vi "RunTest.vi"(8 "error in":errorcluster, 11 "Prueba31 in":refnum<class "Prueba031.lvclass">) -> (0 "error out":errorcluster, 2 "Resultado":string, 3 "Prueba31 out":refnum<class "Prueba031.lvclass">)   [LabVIEW 2019, in "Prueba031.lvclass"]
uses:
  Prueba031.lvclass
  Prueba031.lvclass/Prueba031.ctl
  <vilib>/Utility/miscctls.llb/LVRowAndColumnTypeDef.ctl
  QMH/Message Queue/Enqueue Message (Single).vi
  <vilib>/Utility/error.llb/Error Cluster From Error Code.vi
  RerenceAllControlsToolkit/_get control reference by name.vi
  <vilib>/ErrorRing/Error Ring.xnode
  QMH/Message Queue/Message Queue.lvlib
  QMH/User Event - Stop/User Event - Stop.lvlib
panel:
  in  "Tab":enum32{"externo", "interno"}(tab)
  out "Pict RingB_Ext":u16(ring)
  out "curva_referencia_Ext":dbl
  in  "cb_frec_Ext":string(combo)="63"
  in  "boton_generar_Ext":bool
  out "cumple_Ext":bool
  out "no_cumple_Ext":bool
  in  "seguir_Ext":bool
  out "voltaje_Ext":dbl format="%_3f"
  out "frecuencia_Ext":dbl format="%.2f"
  out "tipo generador_Ext":string
  out "Pict RingA_Ext":u16(ring)
  in  "Tabla_Ext":string[][](table)=[["63"], ["125"], ["250"], ["500"], ["1000"], ["2000"], ["4000"], ["8000"]]
  out "cumple_Int":bool
  out "no_cumple_Int":bool
  in  "seguir_Int":bool
  out "tipo generador_Int":string
  out "Pict RingA_Int":u16(ring)
  out "Pict RingB_Int":u16(ring)
  in  "Tabla_Int":string[][](table)
  # "Vienen de base de datos\nambos\ncambiar a numerico indicador"
  # "Cumple"
  # "No Cumple"
  # "Ponderación C"
  # "Curva de Referencia"
  # "Frecuencia"
  # "3. Ensayo con ponderación frecuencial C con señales acústicas. IEC 61672-3:2006 Cláusula 11"
  # "Monitoreo"
  # "Frecuencia"
  # "Hz"
  # "Voltaje"
  # "V"
  # "Cumple"
  # "No Cumple"
  # "Ponderación C"
  # "3. Ensayo con ponderación frecuencial C con señales acústicas. IEC 61672-3:2006 Cláusula 11"
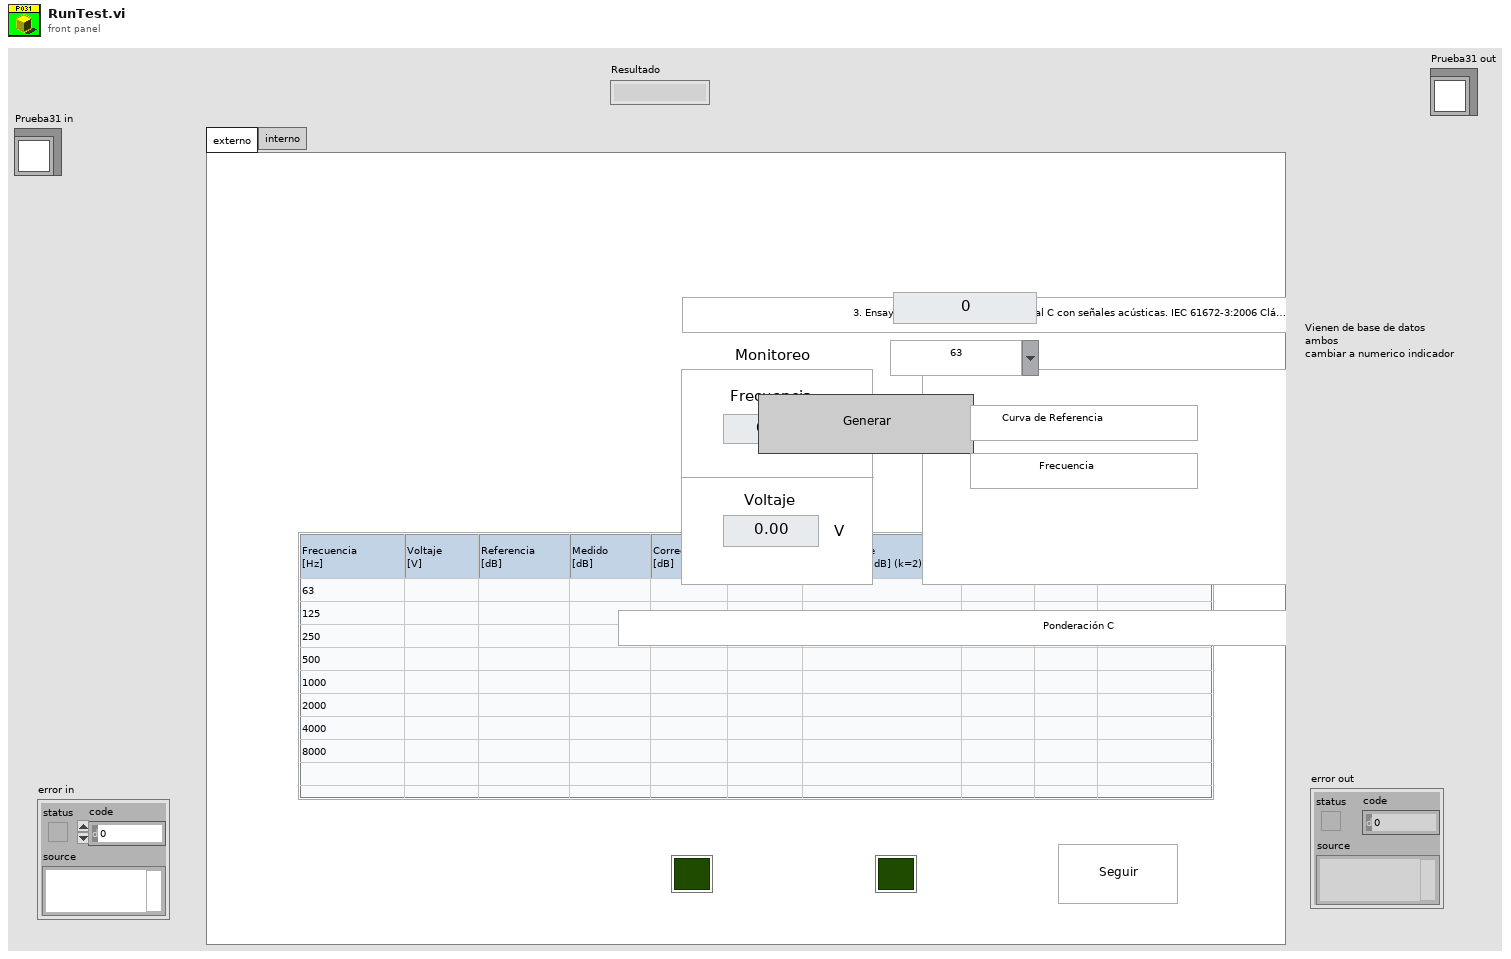
[diagram p1: front panel]
types:
  T1 = typedef "Message Queue.lvlib/All Message Queues.ctl" = cluster{"MHL":refnum<queue>, "Inst_CNT90":refnum<queue>, "Inst_DS360":refnum<queue>, "Inst_Keithley2002":refnum<queue>, "Inst_DAQ":refnum<queue>, "BD":refnum<queue>, "Pistofono":refnum<queue>, "Nexus":refnum<queue>}
  T2 = typedef "LVRowAndColumnTypeDef.ctl" = cluster{"Row":i32, "Column":i32}
  T3 = cluster{"ControlName":string, "ControlReference":refnum<vi>}[]
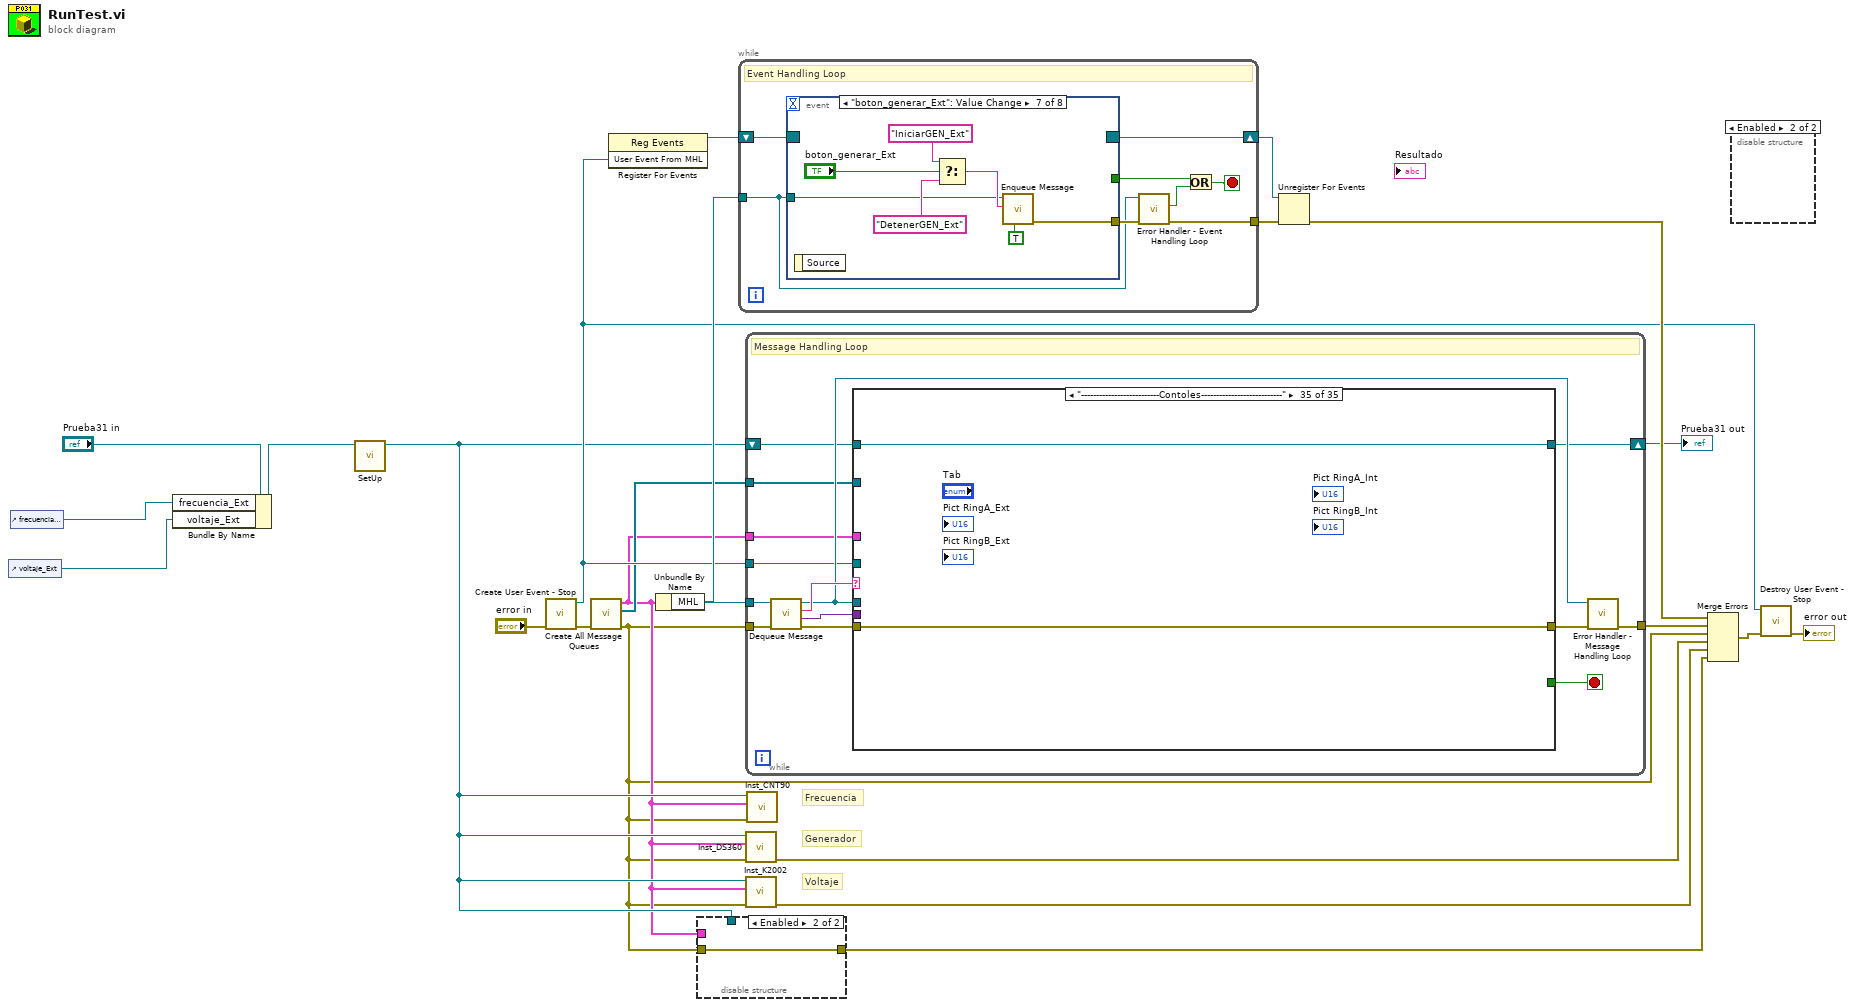
[diagram p0: block diagram]
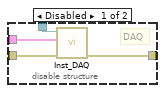
[diagram p2: hidden frame]
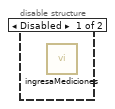
[diagram p3: hidden frame]
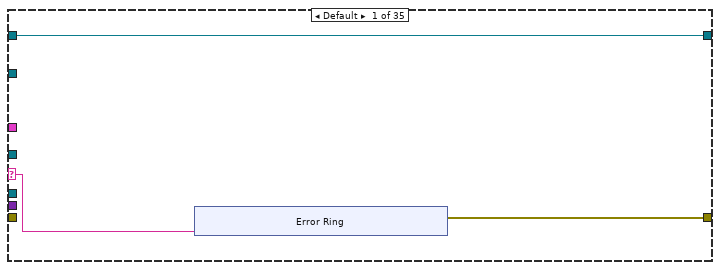
[diagram p4: hidden frame]
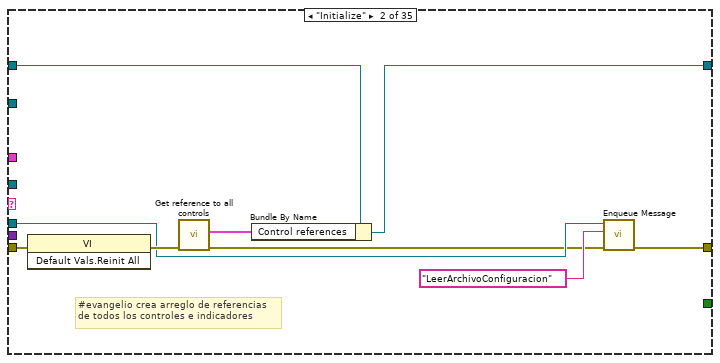
[diagram p5: hidden frame]
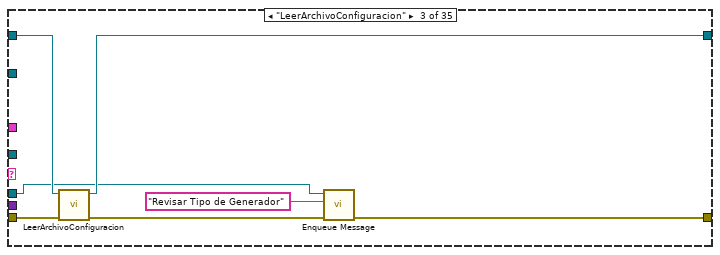
[diagram p6: hidden frame]
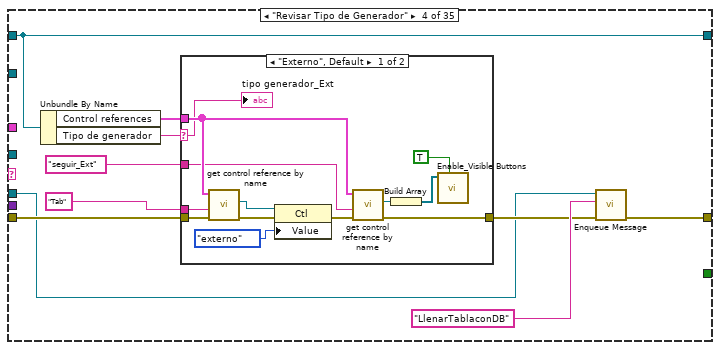
[diagram p7: hidden frame]
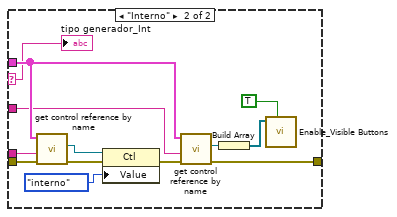
[diagram p8: hidden frame]
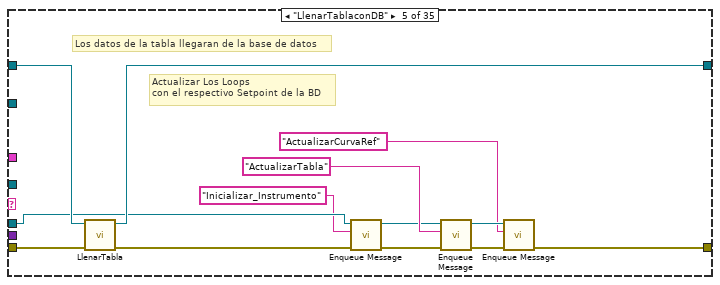
[diagram p9: hidden frame]
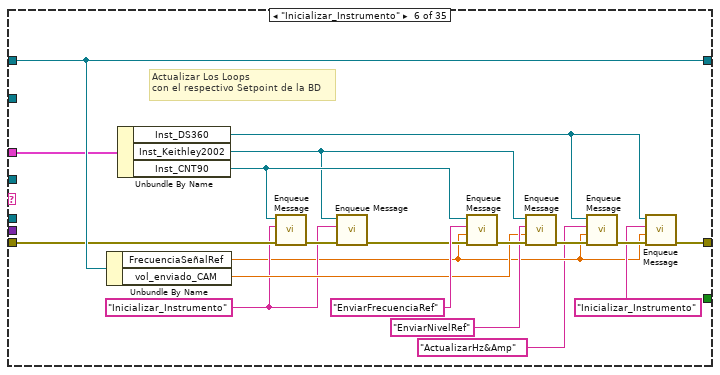
[diagram p10: hidden frame]
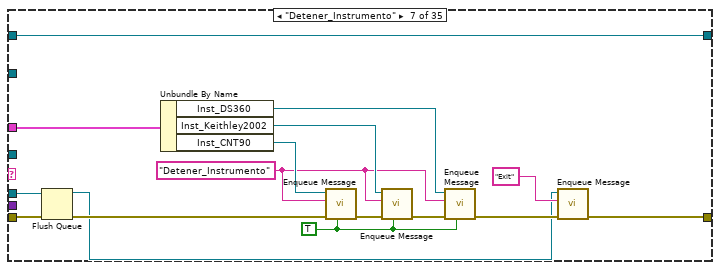
[diagram p11: hidden frame]
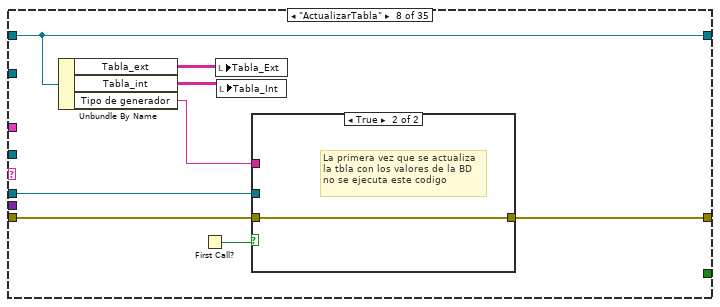
[diagram p12: hidden frame]
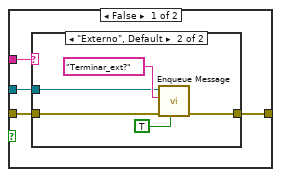
[diagram p13: hidden frame]
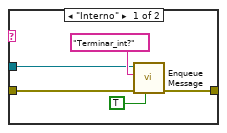
[diagram p14: hidden frame]
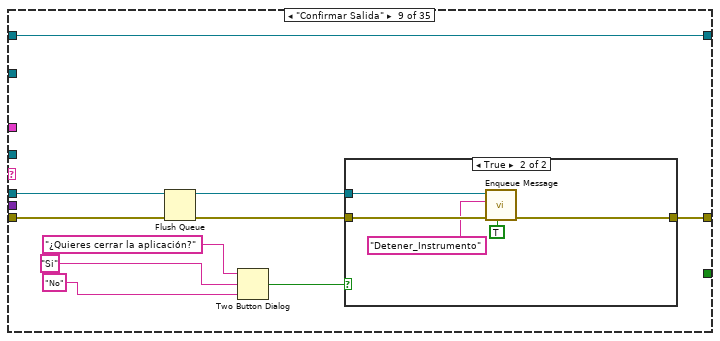
[diagram p15: hidden frame]
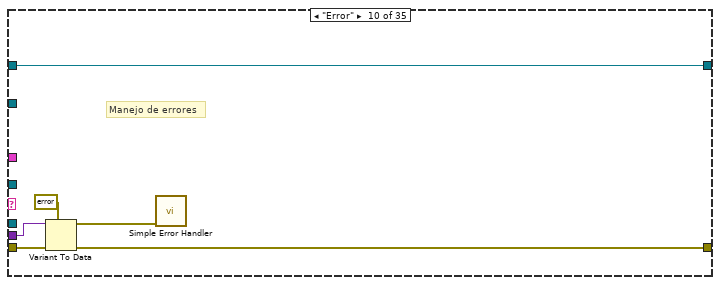
[diagram p17: hidden frame]
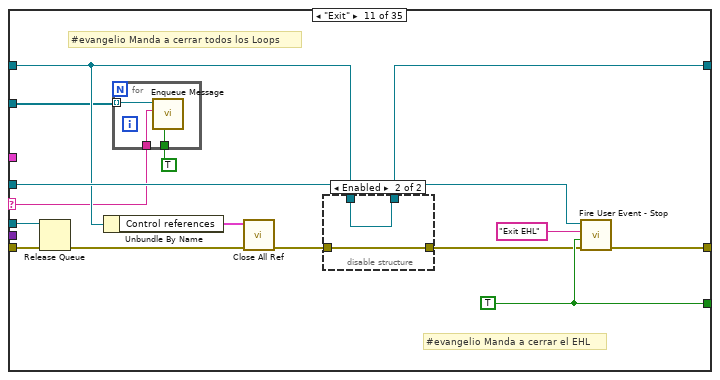
[diagram p18: hidden frame]
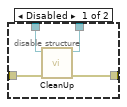
[diagram p19: hidden frame]
diagram:
  # "Voltaje"
  # "Generador"
  # "Frecuencia"
  n1 = control-ref of="voltaje_Ext"() -> (w1:refnum<vi>)
  n2 = control-ref of="frecuencia_Ext"() -> (w2:refnum<vi>)
  n3 = Bundle By Name(cluster="Prueba31 in", "frecuencia_Ext"=w2, "voltaje_Ext"=w1) -> (w3:refnum<class "Prueba031.lvclass">)
  n4 = call-dynamic "SetUp.vi"("Prueba03 in"=w3) -> ("Prueba03 out"=w6:refnum<class "Prueba031.lvclass">)  [unwired: 9 in, 1 out]
  n5 = call "Create User Event - Stop.vi"("error in (no error)"="error in") -> ("error out"=w20:errorcluster, "User Event From MHL"=w14:refnum<user-event>)  [unwired: 9 in]
  n6 = call "Create All Message Queues.vi"("error in (no error)"=w20) -> ("error out"=w4:errorcluster, "PL Queues Array"=w9:refnum<queue>[], "All Message Queues out"=w5:T1)  [unwired: 8 in]
  n7 = register-events(w14) -> (reference out=w23:refnum<event-registration>)  [unwired: 2 in, 1 out]
  n8 = Unbundle By Name(w5) -> ("MHL"=w19:refnum<queue>)
  n9 = disable-structure shown="Enabled" {
    disable-tunnel: w5 -> [w27 _]
    disable-tunnel: w4 -> [w26 w28]
    disable-tunnel: [w25 w28] -> w8
    disable-tunnel: w6 -> [w24 _]
    frame Disabled {
      # "DAQ"
      n10 = call "Inst_DAQ.vi"("error in"=w26, "All Message Queues in"=w27, "Prueba31 in"=w24) -> ("error out"=w25:errorcluster)  [unwired: 8 in]
    }
    frame Enabled {
    }
  }
  n11 = while {
    tunnel: w19 -> [w29]
    tunnel: [w33] -> w22
    shift-right: [w35] -> w21
    shift-left: w23 -> [w36]
    stop <- w30 stop-if-true
    # "Event Handling Loop"
    n12 = event shown="[6] \"boton_generar_Ext\": Value Change" {
      selector: w36 -> [_ _ _ _ _ _ _ _]
      dyn-events: [_ _ _ _ _ _ _ _] -> w35
      timeout: _ -> [_ _ _ _ _ _ _ _]
      tunnel: w29 -> [w39 _ w50 w53 w59 w63 w70 w77]
      tunnel: [w40 _ w47 w54 w61 w68 w75 w78] -> w34
      tunnel: [_ w41 _ _ _ _ _ _] -> w31
      event Panel Close? {
        w37 = TRUE
        n13 = event-data() -> ()  [unwired: 1 in, 1 out]
        n14 = call-poly "Enqueue Message.vi"("Priority Message? (F)"=w37, "Message"="Confirmar Salida", "Message Queue"=w39) -> ("error out"=w40:errorcluster)  [unwired: 7 in, 1 out]
        n15 = event-data("Discard?"=w37) -> ()  [unwired: 1 in, 1 out]
      }
      event User Event {
        n16 = event-data() -> ("User Event"=w43:string, "Event Data"=w42:variant)  [unwired: 1 in]
        n17 = case shown="\"Exit EHL\"" w43 {
          tunnel: w42 -> [_ w45]
          tunnel: [_ w44] -> w41
          frame Default {
          }
          frame "Exit EHL" {
            # "#evangelio Termina\nla ejecucion del EHL"
            n18 = Variant To Data(type=TRUE, Variant=w45) -> (data=w44:bool)  [unwired: 1 in, 1 out]
          }
        }
      }
      event "seguir_Ext": Value Change {
        n19 = event-data() -> ()  [unwired: 1 in, 1 out]
        n20 = call-poly "Enqueue Message.vi"("Priority Message? (F)"=TRUE, "Message"="Detener_Instrumento", "Message Queue"=w50) -> ("error out"=w47:errorcluster)  [unwired: 7 in, 1 out]
      }
      event "seguir_Int": Value Change {
        n21 = event-data() -> ()  [unwired: 1 in, 1 out]
        n22 = call-poly "Enqueue Message.vi"("Priority Message? (F)"=TRUE, "Message"="Exit", "Message Queue"=w53) -> ("error out"=w54:errorcluster)  [unwired: 7 in, 1 out]
      }
      event "Tabla_Ext": Value Change {
        n23 = event-data() -> ()  [unwired: 1 in, 1 out]
        n24 = property on="Tabla_Ext" class="Tbl (strict)"() -> ("Selection Start"=w55:T2)  [unwired: 2 in, 2 out]
        n25 = call-poly "Enqueue Message.vi"("Message"="ActualizarTablaDatoUsuarioExt", "Message Queue"=w59) -> ("error out"=w56:errorcluster, "dup Message Queue"=w58:refnum<queue>)  [unwired: 8 in]
        n26 = call-poly "Enqueue Message.vi"("error in (no error)"=w56, "Message Data"=w55, "Message"="Evaluacion_Ext", "Message Queue"=w58) -> ("error out"=w61:errorcluster)  [unwired: 6 in, 1 out]
      }
      event "Tabla_Int": Value Change {
        n27 = event-data() -> ()  [unwired: 1 in, 2 out]
        n28 = property on="Tabla_Int" class="Tbl (strict)"() -> ("Selection Start"=w66:T2)  [unwired: 2 in, 2 out]
        n29 = call-poly "Enqueue Message.vi"("Message"="ActualizarTablaDatoUsuarioInt", "Message Queue"=w63) -> ("error out"=w65:errorcluster, "dup Message Queue"=w64:refnum<queue>)  [unwired: 8 in]
        n30 = call-poly "Enqueue Message.vi"("error in (no error)"=w65, "Message Data"=w66, "Message"="Evaluacion_Int", "Message Queue"=w64) -> ("error out"=w68:errorcluster)  [unwired: 6 in, 1 out]
      }
      event "boton_generar_Ext": Value Change {
        n31 = event-data() -> ()  [unwired: 1 in, 1 out]
        n32 = Select(t="IniciarGEN_Ext" ("Message"), s="boton_generar_Ext", f="DetenerGEN_Ext" ("Message")) -> (s? t:f=w73:string)
        n33 = call-poly "Enqueue Message.vi"("Priority Message? (F)"=TRUE, "Message"=w73, "Message Queue"=w70) -> ("error out"=w75:errorcluster)  [unwired: 7 in, 1 out]
      }
      event "cb_frec_Ext": Value Change {
        (unwired) "ActualizarCurvaRef" ("Message")
        n34 = event-data() -> ()  [unwired: 1 in, 1 out]
        n35 = call-poly "Enqueue Message.vi"("Message"="NuevoValorFrecuencia", "Message Queue"=w77) -> ("error out"=w78:errorcluster)  [unwired: 8 in, 1 out]
      }
    }
    n36 = call "Error Handler - Event Handling Loop.vi"("error in (no error)"=w34, "Message Queue"=w29) -> ("dup error in"=w33:errorcluster, "Error?"=w32:bool)  [unwired: 7 in, 1 out]
    n37 = Or(x=w31, y=w32) -> (x .or. y?=w30:bool)
  }
  n38 = while {
    tunnel: w4 -> [w92]
    tunnel: w19 -> [w91]
    tunnel: [w85] -> w17
    shift-right: [w83] -> w15
    shift-left: w6 -> [w84]
    tunnel: w5 -> [w81]
    tunnel: w14 -> [w80]
    tunnel: w9 -> [w79]
    stop <- w82 stop-if-true
    # "Message Handling Loop"
    n39 = call "Dequeue Message.vi"("error in (no error)"=w92, "Message Queue"=w91) -> ("error out"=w88:errorcluster, "Message Data"=w89:variant, "Message"=w90:string, "dup Message Queue"=w87:refnum<queue>)  [unwired: 6 in]
    n40 = case shown="\"--------------------------Contoles---------------------------\"" w90 {
      selector: w90 -> [w94 _ _ _ _ _ _ _ _ _ w249 _ _ _ _ _ _ _ _ _ w374 w383 _ _ _ _ _ _ _ _ _ _ _ _ _]
      tunnel: w87 -> [_ w106 w113 w119 w157 _ w190 w205 w226 _ w260 _ _ w278 w293 w303 w328 _ _ _ w369 _ w395 w412 _ w442 _ w464 w476 _ _ w490 w507 _ _]
      tunnel: w89 -> [_ _ _ _ _ _ _ _ _ w242 _ _ _ _ _ _ _ w343 w351 w354 w380 w390 w407 _ _ _ _ _ _ _ _ w502 _ _ _]
      tunnel: w88 -> [_ w111 w118 w125 w167 w178 w194 w206 w233 w243 w259 w272 w276 w285 w296 w306 w329 w344 w352 w355 w381 w391 w408 w421 w437 w446 w461 w471 w480 w483 w487 w503 w516 w532 w537]
      tunnel: [w93 w107 w114 w120 w160 w172 w189 w204 w232 w244 w257 w272 w276 w291 w295 w305 w320 w345 w353 w356 w378 w387 w399 w415 w437 w443 w457 w469 w479 w483 w487 w493 w510 w532 w537] -> w86
      tunnel: w84 -> [w95 w109 w117 w124 w166 w186 w201 w209 w234 w246 w250 w271 w274 w286 w300 w310 w334 w346 w349 w357 w382 w392 w403 w417 w433 w445 w460 w472 w481 w482 w485 w498 w512 w528 w536]
      tunnel: [w95 w108 w116 w124 w163 w186 w201 w209 w234 w246 w251 w271 w275 w286 w300 w310 w335 w346 w350 w357 w382 w392 w410 w417 w433 w445 w460 w467 w481 w482 w486 w505 w512 w528 w536] -> w83
      tunnel: [_ _ _ _ _ _ _ _ _ _ w254 _ _ _ _ _ _ _ _ _ _ _ _ _ _ _ _ _ _ _ _ _ _ _ _] -> w82
      tunnel: w81 -> [_ _ _ _ _ w184 w192 _ _ _ _ _ _ w292 w302 w312 w322 _ _ _ w377 w385 _ _ _ _ _ _ _ _ _ _ _ _ _]
      tunnel: w80 -> [_ _ _ _ _ _ _ _ _ _ w256 _ _ _ _ _ _ _ _ _ _ _ _ _ _ _ _ _ _ _ _ _ _ _ _]
      tunnel: w79 -> [_ _ _ _ _ _ _ _ _ _ w247 _ _ _ _ _ _ _ _ _ _ _ _ _ _ _ _ _ _ _ _ _ _ _ _]
      frame Default {
        n41 = xnode "Error Ring"("parameter 0"=w94) -> ("error out"=w93:errorcluster)
      }
      frame "Initialize" {
        # "#evangelio crea arreglo de referencias\nde todos los controles e indicadores"
        n42 = invoke class="VI" method="Default Vals.Reinit All"(error in=w111) -> (error out=w110:errorcluster)  [unwired: 2 in, 2 out]
        n43 = call "Get reference to all controls.vi"("error in (no error)"=w110) -> ("error out"=w103:errorcluster, "Control references"=w104:T3)  [unwired: 5 in]
        n44 = Bundle By Name(cluster=w109, "Control references"=w104) -> (w108:refnum<class "Prueba031.lvclass">)
        n45 = call-poly "Enqueue Message.vi"("error in (no error)"=w103, "Message"="LeerArchivoConfiguracion", "Message Queue"=w106) -> ("error out"=w107:errorcluster)  [unwired: 7 in, 1 out]
      }
      frame "LeerArchivoConfiguracion" {
        n46 = call "LeerArchivoConfiguracion.vi"("error in"=w118, "Prueba31 in"=w117) -> ("error out"=w115:errorcluster, "Prueba31 out"=w116:refnum<class "Prueba031.lvclass">)  [unwired: 8 in]
        n47 = call-poly "Enqueue Message.vi"("error in (no error)"=w115, "Message"="Revisar Tipo de Generador", "Message Queue"=w113) -> ("error out"=w114:errorcluster)  [unwired: 7 in, 1 out]
      }
      frame "Revisar Tipo de Generador" {
        n48 = Unbundle By Name(w124) -> ("Control references"=w127:T3, "Tipo de generador"=w128:string)
        n49 = case shown="\"Externo\", Default" w128 {
          selector: w128 -> [w129 w142]
          tunnel: w125 -> [w141 w154]
          tunnel: w127 -> [w136 w149]
          tunnel: "Tab" -> [w140 w153]
          tunnel: "seguir_Ext" -> [w134 w147]
          tunnel: [w131 w144] -> w121
          frame "Externo", Default {
            n50 = call-poly "get control reference by name.vi"("error in (no error)"=w141, "Control name"=w140, "Control references"=w136) -> ("error out"=w138:errorcluster, "Ctl Refnum"=w139:refnum<vi>)  [unwired: 3 in]
            n51 = property class="Ctl"(reference=w139, error in=w138, "Value"=enum32{"externo", "interno"}."externo" ("Tab Control")) -> (error out=w135:errorcluster)  [unwired: 1 out]
            n52 = call-poly "get control reference by name.vi"("error in (no error)"=w135, "Control name"=w134, "Control references"=w136) -> ("error out"=w131:errorcluster, "Ctl Refnum"=w133:refnum<vi>)  [unwired: 3 in]
            n53 = Build Array(w133) -> (w132:refnum<vi>[])
            n54 = call "Enable_Visible Buttons.vi"("Enable? (T)"=TRUE, "Controls Ref Array"=w132) -> ()  [unwired: 10 in]
            "tipo generador_Ext" <- w129
          }
          frame "Interno" {
            n55 = call-poly "get control reference by name.vi"("error in (no error)"=w154, "Control name"=w153, "Control references"=w149) -> ("error out"=w151:errorcluster, "Ctl Refnum"=w152:refnum<vi>)  [unwired: 3 in]
            n56 = property class="Ctl"(reference=w152, error in=w151, "Value"=enum32{"externo", "interno"}."interno" ("Tab Control")) -> (error out=w148:errorcluster)  [unwired: 1 out]
            n57 = call-poly "get control reference by name.vi"("error in (no error)"=w148, "Control name"=w147, "Control references"=w149) -> ("error out"=w144:errorcluster, "Ctl Refnum"=w146:refnum<vi>)  [unwired: 3 in]
            n58 = Build Array(w146) -> (w145:refnum<vi>[])
            n59 = call "Enable_Visible Buttons.vi"("Enable? (T)"=TRUE, "Controls Ref Array"=w145) -> ()  [unwired: 10 in]
            "tipo generador_Int" <- w142
          }
        }
        n60 = call-poly "Enqueue Message.vi"("error in (no error)"=w121, "Message"="LlenarTablaconDB", "Message Queue"=w119) -> ("error out"=w120:errorcluster)  [unwired: 7 in, 1 out]
      }
      frame "LlenarTablaconDB" {
        # "Actualizar Los Loops\ncon el respectivo Setpoint de la BD"
        # "Los datos de la tabla llegaran de la base de datos"
        n61 = call "LlenarTabla.vi"("error in (no error)"=w167, "Prueba32 in"=w166) -> ("error out"=w165:errorcluster, "Prueba32 out"=w163:refnum<class "Prueba031.lvclass">)  [unwired: 8 in]
        n62 = call-poly "Enqueue Message.vi"("error in (no error)"=w165, "Message"="Inicializar_Instrumento", "Message Queue"=w157) -> ("error out"=w158:errorcluster, "dup Message Queue"=w156:refnum<queue>)  [unwired: 7 in]
        n63 = call-poly "Enqueue Message.vi"("error in (no error)"=w158, "Message"="ActualizarTabla", "Message Queue"=w156) -> ("error out"=w161:errorcluster, "dup Message Queue"=w162:refnum<queue>)  [unwired: 7 in]
        n64 = call-poly "Enqueue Message.vi"("error in (no error)"=w161, "Message"="ActualizarCurvaRef", "Message Queue"=w162) -> ("error out"=w160:errorcluster)  [unwired: 7 in, 1 out]
      }
      frame "Inicializar_Instrumento" {
        w174 = "Inicializar_Instrumento" ("Message")
        # "Actualizar Los Loops\ncon el respectivo Setpoint de la BD"
        n65 = Unbundle By Name(w186) -> ("FrecuenciaSeñalRef"=w169:dbl, "vol_enviado_CAM"=w181:dbl)
        n66 = Unbundle By Name(w184) -> ("Inst_DS360"=w171:refnum<queue>, "Inst_Keithley2002"=w175:refnum<queue>, "Inst_CNT90"=w179:refnum<queue>)
        n67 = call-poly "Enqueue Message.vi"("error in (no error)"=w178, "Message"=w174, "Message Queue"=w179) -> ("error out"=w177:errorcluster)  [unwired: 7 in, 1 out]
        n68 = call-poly "Enqueue Message.vi"("error in (no error)"=w177, "Message"=w174, "Message Queue"=w175) -> ("error out"=w176:errorcluster)  [unwired: 7 in, 1 out]
        n69 = call-poly "Enqueue Message.vi"("error in (no error)"=w176, "Message Data"=w169, "Message"="EnviarFrecuenciaRef", "Message Queue"=w179) -> ("error out"=w185:errorcluster)  [unwired: 6 in, 1 out]
        n70 = call-poly "Enqueue Message.vi"("error in (no error)"=w185, "Message Data"=w181, "Message"="EnviarNivelRef", "Message Queue"=w175) -> ("error out"=w180:errorcluster)  [unwired: 6 in, 1 out]
        n71 = call-poly "Enqueue Message.vi"("error in (no error)"=w180, "Message Data"=w169, "Message"="ActualizarHz&Amp", "Message Queue"=w171) -> ("error out"=w173:errorcluster)  [unwired: 6 in, 1 out]
        n72 = call-poly "Enqueue Message.vi"("error in (no error)"=w173, "Message Data"=w169, "Message"="Inicializar_Instrumento", "Message Queue"=w171) -> ("error out"=w172:errorcluster)  [unwired: 6 in, 1 out]
      }
      frame "Detener_Instrumento" {
        w195 = TRUE ("Priority Message? (F)")
        w196 = "Detener_Instrumento" ("Message")
        n73 = Flush Queue(queue=w190, error in (no error)=w194) -> (queue out=w187:refnum<queue>, error out=w191:errorcluster)  [unwired: 1 out]
        n74 = Unbundle By Name(w192) -> ("Inst_DS360"=w197:refnum<queue>, "Inst_Keithley2002"=w198:refnum<queue>, "Inst_CNT90"=w200:refnum<queue>)
        n75 = call-poly "Enqueue Message.vi"("Priority Message? (F)"=w195, "error in (no error)"=w191, "Message"=w196, "Message Queue"=w200) -> ("error out"=w199:errorcluster)  [unwired: 6 in, 1 out]
        n76 = call-poly "Enqueue Message.vi"("Priority Message? (F)"=w195, "error in (no error)"=w199, "Message"=w196, "Message Queue"=w198) -> ("error out"=w193:errorcluster)  [unwired: 6 in, 1 out]
        n77 = call-poly "Enqueue Message.vi"("Priority Message? (F)"=w195, "Message"=w196, "Message Queue"=w197) -> ()  [unwired: 7 in, 2 out]
        n78 = call-poly "Enqueue Message.vi"("error in (no error)"=w193, "Message"="Exit", "Message Queue"=w187) -> ("error out"=w189:errorcluster)  [unwired: 7 in, 1 out]
      }
      frame "ActualizarTabla" {
        n79 = Unbundle By Name(w209) -> ("Tabla_ext"=w208:string[][], "Tabla_int"=w207:string[][], "Tipo de generador"=w203:string)
        n80 = First Call?() -> (First Call?: T/F=w202:bool)
        n81 = local write "Tabla_Ext"(w208) -> ()
        n82 = local write "Tabla_Int"(w207) -> ()
        n83 = case shown="True" w202 {
          tunnel: w206 -> [w213 w224]
          tunnel: w205 -> [w212 _]
          tunnel: [w211 w224] -> w204
          tunnel: w203 -> [w210 _]
          frame False {
            n84 = case shown="\"Externo\", Default" w210 {
              tunnel: w213 -> [w216 w222]
              tunnel: w212 -> [w217 w221]
              tunnel: [w215 w220] -> w211
              frame "Interno" {
                n85 = call-poly "Enqueue Message.vi"("Priority Message? (F)"=TRUE, "error in (no error)"=w216, "Message"="Terminar_int?", "Message Queue"=w217) -> ("error out"=w215:errorcluster)  [unwired: 6 in, 1 out]
              }
              frame "Externo", Default {
                n86 = call-poly "Enqueue Message.vi"("Priority Message? (F)"=TRUE, "error in (no error)"=w222, "Message"="Terminar_ext?", "Message Queue"=w221) -> ("error out"=w220:errorcluster)  [unwired: 6 in, 1 out]
              }
            }
          }
          frame True {
            # "La primera vez que se actualiza\nla tbla con los valores de la BD\nno se ejecuta este codigo"
          }
        }
      }
      frame "Confirmar Salida" {
        n87 = Flush Queue(queue=w226, error in (no error)=w233) -> (queue out=w225:refnum<queue>, error out=w227:errorcluster)  [unwired: 1 out]
        n88 = Two Button Dialog(message="¿Quieres cerrar la aplicación?", 1:"No" ("T button name (\"OK\")"), 2:"Si" ("T button name (\"OK\")")) -> (T button?=w228:bool)
        n89 = case shown="True" w228 {
          tunnel: w227 -> [w235 w240]
          tunnel: [w235 w237] -> w232
          tunnel: w225 -> [_ w238]
          frame False {
          }
          frame True {
            n90 = call-poly "Enqueue Message.vi"("Priority Message? (F)"=TRUE, "error in (no error)"=w240, "Message"="Detener_Instrumento", "Message Queue"=w238) -> ("error out"=w237:errorcluster)  [unwired: 6 in, 1 out]
          }
        }
      }
      frame "Error" {
        # "Manejo de errores"
        n91 = Variant To Data(error in=w243, type=errorcluster {"status"=FALSE, "code"=0, "source"=""} ("error constant"), Variant=w242) -> (data=w241:errorcluster, error out=w244:errorcluster)
        n92 = call <vilib>:"Simple Error Handler.vi"("error in (no error)"=w241) -> ()  [unwired: 4 in, 5 out]
      }
      frame "Exit" {
        w254 = TRUE
        # "#evangelio Manda a cerrar el EHL"
        # "#evangelio Manda a cerrar todos los Loops"
        n93 = Release Queue(queue=w260, error in (no error)=w259) -> (error out=w258:errorcluster)  [unwired: 1 in, 2 out]
        n94 = Unbundle By Name(w250) -> ("Control references"=w261:T3)
        n95 = for {
          tunnel: w247 -> [w270] mode=indexing
          tunnel: w249 -> [w269]
          tunnel: TRUE -> [w268]
          n96 = call-poly "Enqueue Message.vi"("Priority Message? (F)"=w268, "Message"=w269, "Message Queue"=w270) -> ()  [unwired: 7 in, 2 out]
        }
        n97 = call "Close All Ref.vi"("error in (no error)"=w258, "Control references"=w261) -> ("error out"=w253:errorcluster)  [unwired: 9 in]
        n98 = disable-structure shown="Enabled" {
          disable-tunnel: w253 -> [w265 w266]
          disable-tunnel: [w264 w266] -> w252
          disable-tunnel: [w263 w267] -> w251
          disable-tunnel: w250 -> [w262 w267]
          frame Disabled {
            n99 = call-dynamic "CleanUp.vi"("error in (no error)"=w265, "Prueba08 in"=w262) -> ("error out"=w264:errorcluster, "Prueba08 out"=w263:refnum<class "Prueba031.lvclass">)  [unwired: 8 in]
          }
          frame Enabled {
          }
        }
        n100 = call "Fire User Event - Stop.vi"("error in (no error)"=w252, "Event Data"=w254, "User Event"="Exit EHL", "User Event in"=w256) -> ("error out"=w257:errorcluster)  [unwired: 7 in]
      }
      frame "---- EXT ----" {
      }
      frame "ActualizarTablaDatoUsuarioExt" {
        n101 = Bundle By Name(cluster=w274, "Tabla_ext"="Tabla_Ext") -> (w275:refnum<class "Prueba031.lvclass">)
      }
      frame "IniciarGEN_Ext" {
        n102 = Unbundle By Name(w286) -> ("Control references"=w287:T3)
        n103 = call-poly "get control reference by name.vi"("error in (no error)"=w285, "Control name"="seguir_ext", "Control references"=w287) -> ("error out"=w281:errorcluster, "Ctl Refnum"=w289:refnum<vi>)  [unwired: 3 in]
        n104 = Build Array(w289) -> (w288:refnum<vi>[])
        n105 = call "Enable_Visible Buttons.vi"("Enable? (T)"=FALSE, "Controls Ref Array"=w288) -> ()  [unwired: 10 in]
        n106 = Unbundle By Name(w292) -> ("Inst_DS360"=w283:refnum<queue>)
        n107 = call-poly "Enqueue Message.vi"("Priority Message? (F)"=TRUE, "error in (no error)"=w281, "Message"="Habilitar_Generador", "Message Queue"=w283) -> ("error out"=w280:errorcluster)  [unwired: 6 in, 1 out]
        n108 = call-poly "Enqueue Message.vi"("error in (no error)"=w280, "Message"="Leer_Voltaje", "Message Queue"=w278) -> ("error out"=w291:errorcluster)  [unwired: 7 in, 1 out]
      }
      frame "Leer_Voltaje" {
        n109 = call-poly "Enqueue Message.vi"("error in (no error)"=w296, "Message"="Leer_Frecuencia", "Message Queue"=w293) -> ("error out"=w301:errorcluster)  [unwired: 7 in, 1 out]
        n110 = Unbundle By Name(w302) -> ("Inst_Keithley2002"=w299:refnum<queue>)
        n111 = call-poly "Enqueue Message.vi"("Message"="Leer_Instrumento", "Message Queue"=w299) -> ()  [unwired: 8 in, 2 out]
        n112 = call "Time Delay"("error in (no error)"=w301, "Delay Time (s)"=1.0) -> ("error out"=w295:errorcluster)  [unwired: 9 in]
      }
      frame "Leer_Frecuencia" {
        n113 = call-poly "Enqueue Message.vi"("error in (no error)"=w306, "Message"="Leer_Voltaje", "Message Queue"=w303) -> ("error out"=w311:errorcluster)  [unwired: 7 in, 1 out]
        n114 = Unbundle By Name(w312) -> ("Inst_CNT90"=w309:refnum<queue>)
        n115 = call-poly "Enqueue Message.vi"("Message"="Leer_Instrumento", "Message Queue"=w309) -> ()  [unwired: 8 in, 2 out]
        n116 = call "Time Delay2"("error in (no error)"=w311, "Delay Time (s)"=1.0) -> ("error out"=w305:errorcluster)  [unwired: 9 in]
      }
      frame "DetenerGEN_Ext" {
        w315 = 0.0 ("frecuencia_Ext")
        w327 = 0.0 ("frecuencia_Ext")
        n117 = Unbundle By Name(w334) -> ("Tabla_ext"=w333:string[][], "voltMedido"=w318:dbl, "Control references"=w337:T3)
        n118 = Flush Queue(queue=w328, error in (no error)=w329) -> (queue out=w325:refnum<queue>, error out=w330:errorcluster)  [unwired: 1 out]
        n119 = local write "frecuencia_Ext"(w327) -> ()
        n120 = local write "voltaje_Ext"(w327) -> ()
        n121 = call-poly "get control reference by name.vi"("error in (no error)"=w330, "Control name"="seguir_ext", "Control references"=w337) -> ("error out"=w326:errorcluster, "Ctl Refnum"=w339:refnum<vi>)  [unwired: 3 in]
        n122 = Build Array(w339) -> (w338:refnum<vi>[])
        n123 = Number To Fractional String(use system decimal point (T)=TRUE, number=w318, precision (6)=i16 3) -> (F-format string=w331:string)  [unwired: 1 in]
        n124 = call "Enable_Visible Buttons.vi"("Controls Ref Array"=w338) -> ()  [unwired: 11 in]
        n125 = Unbundle By Name(w322) -> ("Inst_DS360"=w321:refnum<queue>, "Inst_Keithley2002"=w317:refnum<queue>)
        n126 = call "LlenarVoltajeTabla.vi"("Frecuencia"="cb_frec_Ext", "Dato"=w331, "Tabla in"=w333) -> ("Tabla out"=w323:string[][])  [unwired: 8 in]
        n127 = call-poly "Enqueue Message.vi"("error in (no error)"=w326, "Message"="SiguienteFrecuencia" ("Control name"), "Message Queue"=w325) -> ("error out"=w314:errorcluster)  [unwired: 7 in, 1 out]
        n128 = Bundle By Name(cluster=w334, "Tabla_ext"=w323) -> (w335:refnum<class "Prueba031.lvclass">)
        n129 = Flush Queue(queue=w317, error in (no error)=w314) -> (error out=w316:errorcluster)  [unwired: 2 out]
        n130 = local write "Tabla_Ext"(w323) -> ()
        n131 = call-poly "Enqueue Message.vi"("error in (no error)"=w316, "Message"="Dehabilitar_Generador", "Message Queue"=w321) -> ("error out"=w320:errorcluster)  [unwired: 7 in, 1 out]
        n132 = local write "frecuencia_Ext"(w315) -> ()
        n133 = local write "voltaje_Ext"(w315) -> ()
      }
      frame "DatoRecibidoCNT90" {
        n134 = Variant To Data(error in=w344, type=0.0, Variant=w343) -> (data=→"frecuencia_Ext":dbl, error out=w345:errorcluster)
      }
      frame "DatoRecibidoK2002" {
        n135 = Variant To Data(error in=w352, type=0.0, Variant=w351) -> (data=w347:dbl, error out=w353:errorcluster)
        "voltaje_Ext" <- w347
        n136 = Bundle By Name(cluster=w349, "voltMedido"=w347) -> (w350:refnum<class "Prueba031.lvclass">)
      }
      frame "DatoRecibidoDS360" {
        n137 = disable-structure shown="Disabled" {
          disable-tunnel: [w360 w361] -> w356
          disable-tunnel: w355 -> [w359 w361]
          disable-tunnel: w354 -> [w358 _]
          frame Disabled {
            n138 = Variant To Data(error in=w359, Variant=w358) -> (error out=w360:errorcluster)  [unwired: 1 in, 1 out]
          }
          frame Enabled {
          }
        }
      }
      frame "EnviarFrecuenciaRef" {
        w365 = 0.0 ("frecuencia_Ext")
        w373 = TRUE ("Priority Message? (F)")
        # "envía frecuencia al generador"
        n139 = Flush Queue(queue=w369, error in (no error)=w381) -> (error out=w370:errorcluster)  [unwired: 2 out]
        n140 = Variant To Data(error in=w370, type=w374, Variant=w380) -> (data=w379:string, error out=w364:errorcluster)
        n141 = Unbundle By Name(w377) -> ("Inst_Keithley2002"=w366:refnum<queue>, "Inst_DS360"=w375:refnum<queue>, "Inst_CNT90"=w376:refnum<queue>)
        n142 = Fract/Exp String To Number(string=w379) -> (number=w371:dbl)  [unwired: 3 in, 1 out]
        n143 = Flush Queue(queue=w376, error in (no error)=w364) -> (queue out=w367:refnum<queue>, error out=w363:errorcluster)  [unwired: 1 out]
        n144 = Flush Queue(queue=w366, error in (no error)=w363) -> (error out=w362:errorcluster)  [unwired: 2 out]
        n145 = Flush Queue(queue=w375) -> (queue out=w368:refnum<queue>)  [unwired: 1 in, 2 out]
        n146 = call-poly "Enqueue Message.vi"("Priority Message? (F)"=w373, "error in (no error)"=w362, "Message Data"=w371, "Message"=w374, "Message Queue"=w367) -> ("error out"=w378:errorcluster)  [unwired: 5 in, 1 out]
        n147 = local write "frecuencia_Ext"(w365) -> ()
        n148 = local write "voltaje_Ext"(w365) -> ()
        n149 = call-poly "Enqueue Message.vi"("Priority Message? (F)"=w373, "Message Data"=w371, "Message"="ActualizarHz&Amp", "Message Queue"=w368) -> ()  [unwired: 6 in, 2 out]
      }
      frame "EnviarNivelRef" {
        n150 = Variant To Data(error in=w391, type=w383, Variant=w390) -> (data=w389:string, error out=w388:errorcluster)
        n151 = Unbundle By Name(w385) -> ("Inst_Keithley2002"=w384:refnum<queue>)
        n152 = Fract/Exp String To Number(string=w389) -> (number=w386:dbl)  [unwired: 3 in, 1 out]
        n153 = call-poly "Enqueue Message.vi"("error in (no error)"=w388, "Message Data"=w386, "Message"=w383, "Message Queue"=w384) -> ("error out"=w387:errorcluster)  [unwired: 6 in, 1 out]
      }
      frame "Evaluacion_Ext" {
        # "columna"
        n154 = Variant To Data(error in=w408, type=T2 {"Row"=0, "Column"=0} ("Selection Start"), Variant=w407) -> (data=w405:T2, error out=w409:errorcluster)
        n155 = Unbundle By Name(w405) -> ("Row"=w402:i32)  [unwired: 1 out]
        n156 = call "ObtenerDatosdelatabla.vi"("tipo_gen"="externo", "Column"=3, "Row"=w402, "Prueba32 in"=w403) -> ("Prueba32 out"=w404:refnum<class "Prueba031.lvclass">)  [unwired: 7 in]
        n157 = call "cumplimiento_ext.vi"("error in (no error)"=w409, "Prueba08 in"=w404) -> ("error out"=w401:errorcluster, "Prueba08 out"=w410:refnum<class "Prueba031.lvclass">)  [unwired: 7 in, 1 out]
        n158 = Flush Queue(queue=w395, error in (no error)=w401) -> (queue out=w394:refnum<queue>, error out=w396:errorcluster)  [unwired: 1 out]
        n159 = call-poly "Enqueue Message.vi"("Priority Message? (F)"=TRUE, "error in (no error)"=w396, "Message"="ActualizarTabla", "Message Queue"=w394) -> ("error out"=w399:errorcluster)  [unwired: 6 in, 1 out]
      }
      frame "Terminar_ext?" {
        # "si son todos\ndistntos a cero\nentonces todos se\nhan evaluado"
        n160 = Unbundle By Name(w417) -> ("Tabla_ext"=w416:string[][])
        n161 = Index Array(array=w416, index (col)=9 ("disabled index (col)")) -> (element=w419:string[])  [unwired: 1 in]
        n162 = Flush Queue(queue=w412, error in (no error)=w421) -> (queue out=w411:refnum<queue>, error out=w413:errorcluster)  [unwired: 1 out]
        n163 = for {
          tunnel: [w429] -> w418 mode=indexing
          tunnel: w419 -> [w427] mode=indexing
          n164 = Not Equal?(x=w427, y="--") -> (x != y?=w429:bool)
        }
        n165 = And Array Elements(Boolean array=w418) -> (logical AND=w414:bool)
        n166 = case shown="False" w414 {
          tunnel: w413 -> [w422 w426]
          tunnel: [w422 w425] -> w415
          tunnel: w411 -> [_ w424]
          frame False {
          }
          frame True {
            n167 = call-poly "Enqueue Message.vi"("error in (no error)"=w426, "Message"="Cumple_ext?", "Message Queue"=w424) -> ("error out"=w425:errorcluster)  [unwired: 7 in, 1 out]
          }
        }
      }
      frame "Cumple_ext?" {
        # "si todos cumplen\nentonces el ensayo\ncumple"
        n168 = Unbundle By Name(w433) -> ("Tabla_ext"=w432:string[][])
        n169 = Index Array(array=w432, index (col)=9 ("disabled index (col)")) -> (element=w435:string[])  [unwired: 1 in]
        n170 = for {
          tunnel: [w440] -> w434 mode=indexing
          tunnel: w435 -> [w438] mode=indexing
          n171 = Equal?(x=w438, y="Cumple") -> (x = y?=w440:bool)
        }
        n172 = And Array Elements(Boolean array=w434) -> (logical AND=w430:bool)
        "cumple_Ext" <- w430
        n173 = Not(x=w430) -> (.not. x?=→"no_cumple_Ext":bool)
      }
      frame "ActualizarCurvaRef" {
        n174 = disable-structure shown="Enabled" {
          disable-tunnel: w445 -> [w453 w455]
          disable-tunnel: [w447 w454] -> w444
          frame Disabled {
            n175 = Unbundle By Name(w453) -> ("Tabla_ext"=w451:string[][])
            n176 = local read "cb_frec_Ext"() -> (w452:string)
            n177 = call "ObtenerFilaEnUso.vi"("Tabla in"=w451, "Frecuencia"=w452) -> ("index of element"=w450:i32)  [unwired: 9 in]
            n178 = Index Array(array=w451, index (row)=w450, index (col)=1 ("disabled index (col)")) -> (element=w448:string)
            n179 = Fract/Exp String To Number(string=w448) -> (number=w447:dbl)  [unwired: 3 in, 1 out]
          }
          frame Enabled {
            n180 = Unbundle By Name(w455) -> ("NivelSeñalRef"=w454:dbl)
          }
        }
        "curva_referencia_Ext" <- w444
        n181 = call-poly "Enqueue Message.vi"("error in (no error)"=w446, "Message"="ActualizarComboBoxFrecuenciaExt", "Message Queue"=w442) -> ("error out"=w443:errorcluster)  [unwired: 7 in, 1 out]
      }
      frame "ActualizarComboBoxFrecuenciaExt" {
        n182 = Unbundle By Name(w460) -> ("Frecuencias(Hz)"=w459:string[])
        n183 = Index Array(array=w459, index=0) -> (element=w456:string)
        n184 = property on="cb_frec_Ext" class="CmbBox"(error in=w461, "Value"=w456) -> (error out=w457:errorcluster)  [unwired: 1 in, 1 out]
      }
      frame "SiguienteFrecuencia" {
        w462 = 0.0 ("frecuencia_Ext")
        n185 = Flush Queue(queue=w464, error in (no error)=w471) -> (queue out=w463:refnum<queue>, error out=w465:errorcluster)  [unwired: 1 out]
        n186 = call "NuevaFrecuencia.vi"("error in (no error)"=w465, "Prueba031 in"=w472) -> ("error out"=w470:errorcluster, "newFrec"=w466:string, "Prueba031 out"=w467:refnum<class "Prueba031.lvclass">)  [unwired: 7 in]
        n187 = call-poly "Enqueue Message.vi"("error in (no error)"=w470, "Message Data"=w466, "Message"="EnviarFrecuenciaRef", "Message Queue"=w463) -> ("error out"=w469:errorcluster)  [unwired: 6 in, 1 out]
        n188 = local write "frecuencia_Ext"(w462) -> ()
        n189 = local write "voltaje_Ext"(w462) -> ()
      }
      frame "NuevoValorFrecuencia" {
        n190 = Flush Queue(queue=w476, error in (no error)=w480) -> (queue out=w475:refnum<queue>, error out=w477:errorcluster)  [unwired: 1 out]
        n191 = property on="cb_frec_Ext" class="CmbBox"(error in=w477) -> (error out=w474:errorcluster, "Value"=w473:string)  [unwired: 1 in, 1 out]
        n192 = call-poly "Enqueue Message.vi"("error in (no error)"=w474, "Message Data"=w473, "Message"="EnviarFrecuenciaRef", "Message Queue"=w475) -> ("error out"=w479:errorcluster)  [unwired: 6 in, 1 out]
      }
      frame "---- INT ----" {
      }
      frame "ActualizarTablaDatoUsuarioInt" {
        n193 = Bundle By Name(cluster=w485, "Tabla_int"="Tabla_Int") -> (w486:refnum<class "Prueba031.lvclass">)
      }
      frame "Evaluacion_Int" {
        n194 = Variant To Data(error in=w503, type=T2 {"Row"=0, "Column"=0} ("Selection Start"), Variant=w502) -> (data=w500:T2, error out=w504:errorcluster)
        n195 = Unbundle By Name(w500) -> ("Row"=w497:i32)  [unwired: 1 out]
        n196 = call "ObtenerDatosdelatabla.vi"("tipo_gen"="interno", "Column"=2, "Row"=w497, "Prueba32 in"=w498) -> ("Prueba32 out"=w499:refnum<class "Prueba031.lvclass">)  [unwired: 7 in]
        n197 = call "cumplimiento_int.vi"("error in (no error)"=w504, "Prueba08 in"=w499) -> ("error out"=w496:errorcluster, "Prueba08 out"=w505:refnum<class "Prueba031.lvclass">)  [unwired: 7 in, 1 out]
        n198 = Flush Queue(queue=w490, error in (no error)=w496) -> (queue out=w489:refnum<queue>, error out=w491:errorcluster)  [unwired: 1 out]
        n199 = call-poly "Enqueue Message.vi"("Priority Message? (F)"=TRUE, "error in (no error)"=w491, "Message"="ActualizarTabla", "Message Queue"=w489) -> ("error out"=w493:errorcluster)  [unwired: 6 in, 1 out]
      }
      frame "Terminar_int?" {
        # "si son todos\ndistntos a cero\nentonces todos se\nhan evaluado"
        n200 = Unbundle By Name(w512) -> ("Tabla_int"=w511:string[][])
        n201 = Index Array(array=w511, index (col)=8 ("disabled index (col)")) -> (element=w514:string[])  [unwired: 1 in]
        n202 = Flush Queue(queue=w507, error in (no error)=w516) -> (queue out=w506:refnum<queue>, error out=w508:errorcluster)  [unwired: 1 out]
        n203 = for {
          tunnel: [w524] -> w513 mode=indexing
          tunnel: w514 -> [w522] mode=indexing
          n204 = Not Equal?(x=w522, y="--") -> (x != y?=w524:bool)
        }
        n205 = And Array Elements(Boolean array=w513) -> (logical AND=w509:bool)
        n206 = case shown="False" w509 {
          tunnel: w508 -> [w517 w521]
          tunnel: [w517 w520] -> w510
          tunnel: w506 -> [_ w519]
          frame False {
          }
          frame True {
            n207 = call-poly "Enqueue Message.vi"("error in (no error)"=w521, "Message"="Cumple_int?", "Message Queue"=w519) -> ("error out"=w520:errorcluster)  [unwired: 7 in, 1 out]
          }
        }
      }
      frame "Cumple_int?" {
        # "si todos cumplen\nentonces el ensayo\ncumple"
        n208 = Unbundle By Name(w528) -> ("Tabla_int"=w527:string[][])
        n209 = Index Array(array=w527, index (col)=8 ("disabled index (col)")) -> (element=w530:string[])  [unwired: 1 in]
        n210 = for {
          tunnel: [w535] -> w529 mode=indexing
          tunnel: w530 -> [w533] mode=indexing
          n211 = Equal?(x=w533, y="Cumple") -> (x = y?=w535:bool)
        }
        n212 = And Array Elements(Boolean array=w529) -> (logical AND=w525:bool)
        "cumple_Int" <- w525
        n213 = Not(x=w525) -> (.not. x?=→"no_cumple_Int":bool)
      }
      frame "--------------------------Contoles---------------------------" {
      }
    }
    n214 = call "Error Handler - Message Handling Loop.vi"("error in (no error)"=w86, "Message Queue"=w87) -> ("dup error in"=w85:errorcluster)  [unwired: 8 in, 1 out]
  }
  "Prueba31 out" <- w15
  n215 = call "Inst_DS360.vi"("error in"=w4, "All Message Queues in"=w5, "Prueba31 in"=w6) -> ("error out"=w11:errorcluster)  [unwired: 8 in]
  n216 = call "Inst_K2002.vi"("error in"=w4, "All Message Queues in"=w5, "Prueba31 in"=w6) -> ("error out"=w10:errorcluster)  [unwired: 8 in]
  n217 = call "Inst_CNT90.vi"("error in"=w4, "All Message Queues in"=w5, "Prueba031 in"=w6) -> ()  [unwired: 8 in, 1 out]
  n218 = Unregister For Events(event registration refnum=w21, error in=w22) -> (error out=w18:errorcluster)
  n219 = Merge Errors(w18, w17, w4, w11, w10, w8) -> (w16:errorcluster)
  n220 = disable-structure shown="Enabled" {
    frame Disabled {
      n221 = call "ingresaMediciones.vi"() -> ()  [unwired: 10 in, 2 out]
    }
    frame Enabled {
    }
  }
  n222 = call "Destroy User Event - Stop.vi"("error in (no error)"=w16, "User Event"=w14) -> ("error out"=→"error out":errorcluster)  [unwired: 9 in]
